vi "Removefrombd.vi"(10 "TextToDelete":string="sdfdsfsd", 11 "VIRefnum":refnum<vi>) -> (3 "LogicalOR":bool)   [LabVIEW 2021]
uses:
  <vilib>/Utility/traverseref.llb/TRef TravTarget.ctl
  <vilib>/Utility/traverseref.llb/VI Scripting - Traverse.lvlib
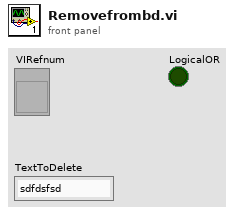
[diagram p1: front panel]
types:
  T1 = typedef "TRef TravTarget.ctl" = enum16{"FP", "BD", "Other"}
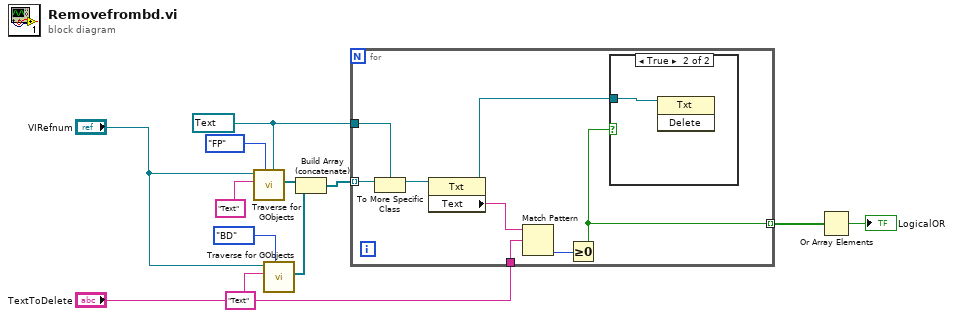
[diagram p0: block diagram]
diagram:
  w9 = refnum<vi> refnum ("Other Refnum")
  n1 = call <vilib>:"Traverse for GObjects.vi"("Other Refnum"=w9, "Traverse Target"=TRef_TravTarget."FP", "Class Name"="Text", "VI Refnum"="VIRefnum") -> ("References"=w10:refnum<vi>[])  [unwired: 4 in, 3 out]
  n2 = call <vilib>:"Traverse for GObjects.vi"("Traverse Target"=TRef_TravTarget."BD", "Class Name"="Text", "VI Refnum"="VIRefnum") -> ("References"=w5:refnum<vi>[])  [unwired: 5 in, 3 out]
  n3 = Build Array (concatenate)(w10, w5) -> (w6:refnum<vi>[])
  n4 = for {
    tunnel: w6 -> [w20] mode=indexing
    tunnel: w9 -> [w18]
    tunnel: [w14] -> w3 mode=indexing
    tunnel: "TextToDelete" -> [w13]
    n5 = To More Specific Class(target class=w18, reference=w20) -> (specific class reference=w19:refnum<vi>)  [unwired: 1 in, 1 out]
    n6 = property class="Txt"(reference=w19) -> (reference out=w15:refnum<vi>, "Text"=w16:string)  [unwired: 1 in, 1 out]
    n7 = Match Pattern(string=w16, regular expression=w13) -> (offset past match=w17:i32)  [unwired: 1 in, 3 out]
    n8 = Greater Or Equal To 0?(x=w17) -> (x >= 0?=w14:bool)
    n9 = case shown="True" w14 {
      tunnel: w15 -> [_ w21]
      frame False {
      }
      frame True {
        n10 = invoke class="Txt" method="Delete"(reference=w21) -> ()  [unwired: 2 in, 3 out]
      }
    }
  }
  n11 = Or Array Elements(Boolean array=w3) -> (logical OR=→"LogicalOR":bool)
